vi "SDK Test.vi"() -> ()   [LabVIEW 2018]
uses:
  <instrlib>/Fujifilm X Series GFX System Digital Camera/Fujifilm X Series GFX System Digital Camera.lvlib
panel:
  out "Found GFX100 Cameras (*USB connected)":i32
  out "Result Detect":i32
  out "Result Init":i32
  out "SDK Version":string
  out "Result SDK Version":i32
  out "Result Exit":i32
  out "error out":errorcluster
  in  "error in (no error)":errorcluster
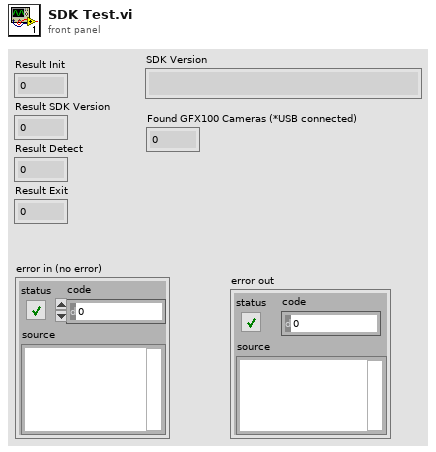
[diagram p1: front panel]
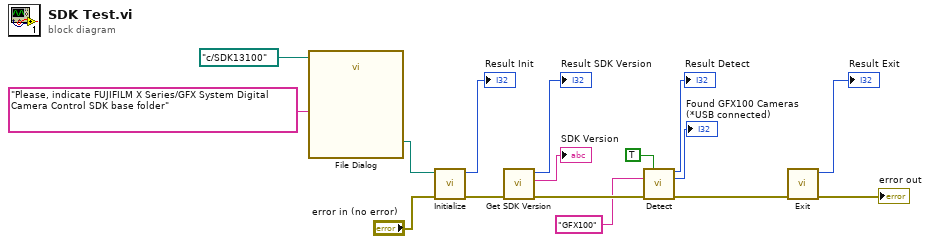
[diagram p0: block diagram]
diagram:
  n1 = call "File Dialog"("start path"=path "c:/SDK13100" ("SDK Directory Path"), "prompt"="Please, indicate FUJIFILM X Series/GFX System Digital Camera Control SDK base folder") -> ("selected path"=w1:path)  [unwired: 10 in, 3 out]
  n2 = call <instrlib>:"Initialize.vi"("error in (no error)"="error in (no error)", "SDK Directory Path"=w1) -> ("error out"=w12:errorcluster, "Result"=→"Result Init":i32)  [unwired: 8 in]
  n3 = call <instrlib>:"Get SDK Version.vi"("error in (no error)"=w12) -> ("error out"=w9:errorcluster, "Version"=→"SDK Version":string, "Result"=→"Result SDK Version":i32)  [unwired: 8 in]
  n4 = call <instrlib>:"Detect.vi"("USB (True)"=TRUE, "DeviceName"="GFX100", "error in (no error)"=w9) -> ("Result"=→"Result Detect":i32, "Count"=→"Found GFX100 Cameras (*USB connected)":i32, "error out"=w8:errorcluster)  [unwired: 10 in]
  n5 = call <instrlib>:"Exit.vi"("error in (no error)"=w8) -> ("error out"=→"error out":errorcluster, "Result"=→"Result Exit":i32)  [unwired: 9 in]
